vi "USB - Write and Read Array of Synchronous Messages.vi"(8 "error in":errorcluster, 10 "Array of Messages to Send":string[](array[string]), 11 "VISA resource name in":refnum<visa-resource-name>) -> (0 "error out":errorcluster, 2 "Received Message Array":string[](array[string]), 3 "VISA resource name out":refnum<visa-resource-name>)   [LabVIEW 2020]
doc: "Sends an array of USB/Serial messages and listens for the response to each message."
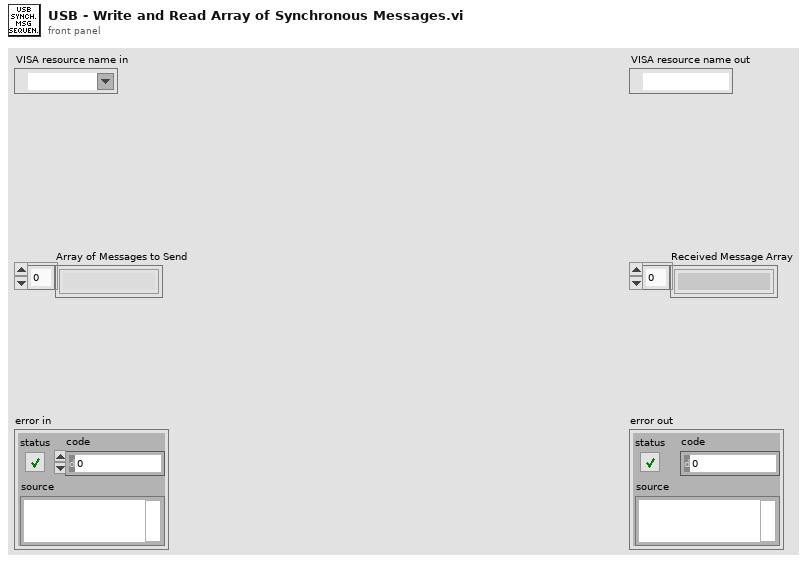
[diagram p1: front panel]
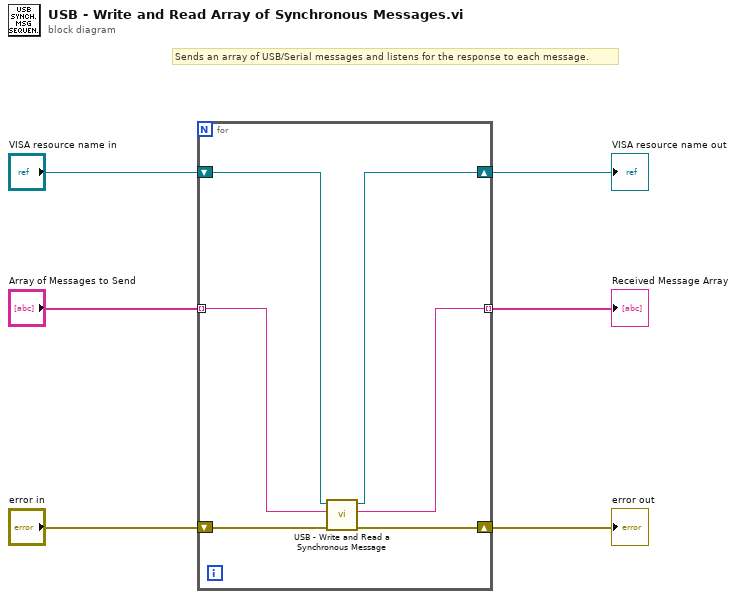
[diagram p0: block diagram]
diagram:
  # "Sends an array of USB/Serial messages and listens for the response to each message."
  n1 = for {
    shift-right: [w11] -> w5
    shift-left: "error in" -> [w12]
    tunnel: "Array of Messages to Send" -> [w8] mode=indexing
    tunnel: [w7] -> w3 mode=indexing
    shift-right: [w10] -> w2
    shift-left: "VISA resource name in" -> [w9]
    n2 = call "USB - Write and Read a Synchronous Message.vi"("error in"=w12, "Message to Send"=w8, "VISA resource name in"=w9) -> ("error out"=w11:errorcluster, "Received Text"=w7:string, "VISA resource name out"=w10:refnum<visa-resource-name>)  [unwired: 6 in]
  }
  "error out" <- w5
  "Received Message Array" <- w3
  "VISA resource name out" <- w2
